vi "FestoCPX.Valves.Reset.vi"(8 "error in":errorcluster) -> (0 "error out":errorcluster)   [LabVIEW 2014]
uses:
  FestoCPX.DO.Data.States.Clear.vi
  FestoCPX.DO.Signal.ctl
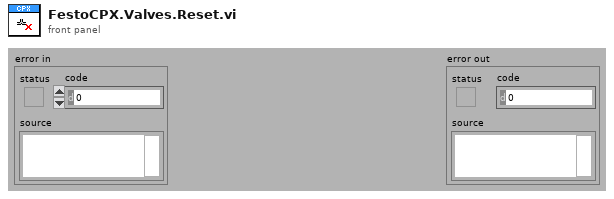
[diagram p1: front panel]
types:
  T1 = typedef "FestoCPX.DO.Signal.ctl" = enum16{"White Button LED", "Red Button LED", "Blue Button LED", "Yellow Button LED", "Safety Circuit Reset", "Air Main Valve", "Laser Interlock", "Laser Shutterlock", "Fume Extraction Unit Start", "Traffic Light Red", "Traffic Light Orange", "Traffic Light Green", "Horn", "Product OK", "Product NOK", "PS OUT Enable", "Q4 Press Work", "Q4 Press Home", "Q5 Electric Conn Work", "Q5 Electric Conn Home", "Q6 Pneumatic and Electric Conn Work", "Q6 Pneumatic and Electric Conn Home", "Q7 Pneumatic Conn Work", "Q7 Pneumatic Conn Home", "Q8 Exhaust Conn Work", "Q8 Exhaust Conn Home", "Q9 Clamp Work", "Q9 Clamp Home", "Q12 Table Turn Work", "Q12 Table Turn Home"}
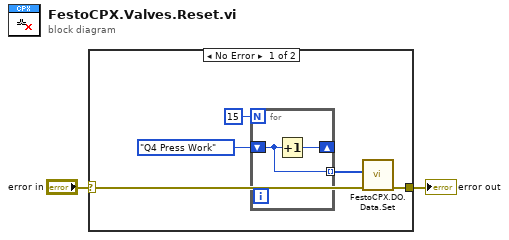
[diagram p0: block diagram]
diagram:
  n1 = case shown="No Error" "error in" {
    selector: "error in" -> [w5 w10]
    tunnel: [w4 w10] -> w2
    frame No Error {
      n2 = for {
        N: 15 -> [_]
        tunnel: [w8] -> w6 mode=indexing
        shift-right: [w9] -> _
        shift-left: FestoCPX.DO.Signal."Q4 Press Work" ("CPX.DO") -> [w8]
        n3 = Increment(x=w8) -> (x+1=w9:T1)
      }
      n4 = call-poly "FestoCPX.DO.Data.Set.vi"("error in (no error)"=w5, "CPX.DO"=w6) -> ("error out"=w4:errorcluster)  [unwired: 9 in]
    }
    frame Error {
    }
  }
  "error out" <- w2
